vi "Overlay XY Position to Coords.vi"(10 "XY":T2(array[cluster]), 11 "Graph":refnum<vi>) -> (2 "Coords":T1(array[cluster]), 3 "Graph out":refnum<vi>)   [LabVIEW 2016]
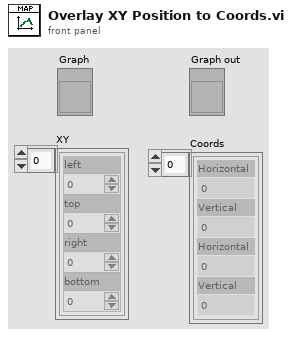
[diagram p1: front panel]
types:
  T1 = cluster{"Horizontal":i32, "Vertical":i32, "Horizontal":i32, "Vertical":i32}[]
  T2 = cluster{"left":dbl, "top":dbl, "right":dbl, "bottom":dbl}[]
  T3 = typedef "LVRectTypeDef.ctl" = cluster{"Left":i16, "Top":i16, "Right":i16, "Bottom":i16}
  T4 = typedef "LVPoint32TypeDef.ctl" = cluster{"Horizontal":i32, "Vertical":i32}
  T5 = cluster{"Horizontal":i32, "Vertical":i32, "Horizontal":i32, "Vertical":i32}
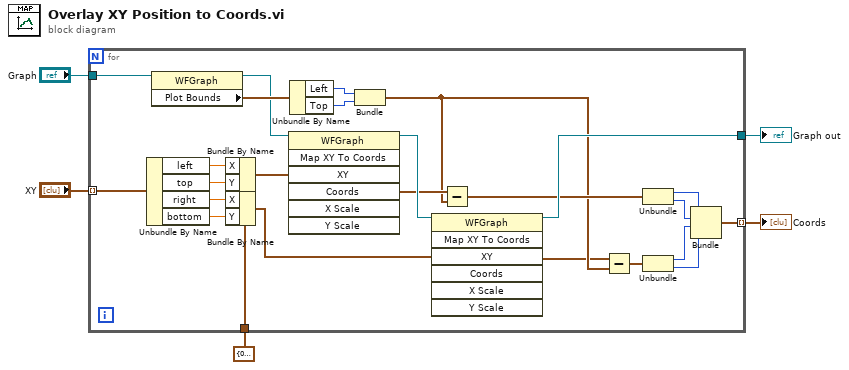
[diagram p0: block diagram]
diagram:
  n1 = for {
    tunnel: "XY" -> [w30] mode=indexing
    tunnel: "Graph" -> [w7]
    tunnel: [w18] -> w3 mode=indexing
    tunnel: [w17] -> w2
    tunnel: cluster{"X":dbl, "Y":dbl} {"X"=0.0, "Y"=0.0} ("XY") -> [w16]
    n2 = Unbundle By Name(w30) -> ("left"=w29:dbl, "top"=w28:dbl, "right"=w27:dbl, "bottom"=w26:dbl)
    n3 = property class="WFGraph"(reference=w7) -> (reference out=w6:refnum<vi>, "Plot Bounds"=w15:T3)  [unwired: 1 in, 1 out]
    n4 = Bundle By Name(cluster=w16, "X"=w29, "Y"=w28) -> (w25:cluster{"X":dbl, "Y":dbl})
    n5 = Bundle By Name(cluster=w16, "X"=w27, "Y"=w26) -> (w23:cluster{"X":dbl, "Y":dbl})
    n6 = invoke class="WFGraph" method="Map XY To Coords"(reference=w6, "XY"=w25) -> (reference out=w24:refnum<vi>, "Coords"=w12:T4)  [unwired: 5 in, 5 out]
    n7 = Unbundle By Name(w15) -> ("Left"=w14:i16, "Top"=w13:i16)
    n8 = Bundle("Left"=w14, "Top"=w13) -> (w10:cluster{"Left":i16, "Top":i16})  [unwired: 1 in]
    n9 = invoke class="WFGraph" method="Map XY To Coords"(reference=w24, "XY"=w23) -> (reference out=w17:refnum<vi>, "Coords"=w9:T4)  [unwired: 5 in, 5 out]
    n10 = Subtract(x=w12, y=w10) -> (x-y=w11:T4)
    n11 = Subtract(x=w9, y=w10) -> (x-y=w8:T4)
    n12 = Unbundle(w11) -> ("Horizontal"=w22:i32, "Vertical"=w21:i32)
    n13 = Unbundle(w8) -> ("Horizontal"=w20:i32, "Vertical"=w19:i32)
    n14 = Bundle("Horizontal"=w22, "Vertical"=w21, "Horizontal"=w20, "Vertical"=w19) -> (w18:T5)  [unwired: 1 in]
  }
  "Coords" <- w3
  "Graph out" <- w2
